vi "Vecto Info JSON.vi"(8 "error in (no error)":errorcluster, 10 "Vecto Info":T1) -> (0 "error out":errorcluster, 2 "JSON string":string)   [LabVIEW 2020, in "Vecto.lvlib" / "InfoController.lvclass"]
uses:
  InfoController.lvclass
  Connection Type.ctl
  Vecto.lvlib
  Connection Info.ctl
  Vecto Info.ctl
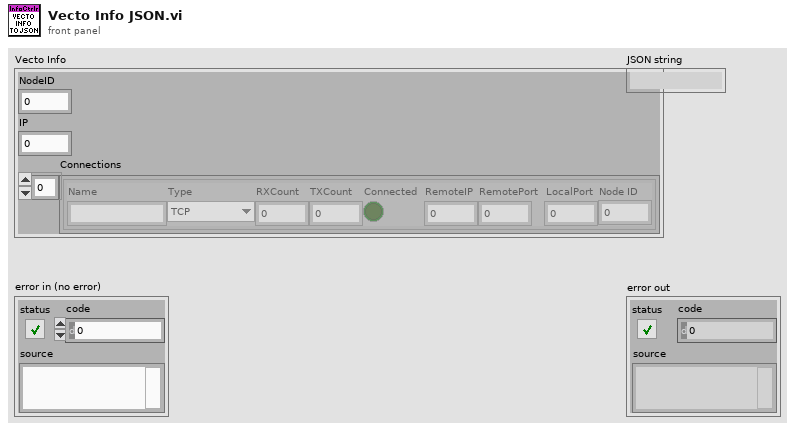
[diagram p1: front panel]
types:
  T1 = typedef "Vecto.lvlib/Vecto Info.ctl" = cluster{"NodeID":i32, "IP":u32, "Connections":T2[]}
  T2 = typedef "Vecto.lvlib/Connection Info.ctl" = cluster{"Name":string, "Type":T3, "RXCount":i32, "TXCount":i32, "Connected":bool, "RemoteIP":u32, "RemotePort":u16, "LocalPort":u16, "Node ID":u32}
  T3 = typedef "Vecto.lvlib/Connection Type.ctl" = enum16{"TCP", "Telemetry", "Discovery", "HTTP"}
  T4 = cluster{"Name":string, "Type":string, "RXCount":i32, "TXCount":i32, "Connected":bool, "RemoteIP":u32, "RemotePort":u16, "LocalPort":u16}[]
  T5 = cluster{"Name":string, "Type":string, "RXCount":i32, "TXCount":i32, "Connected":bool, "RemoteIP":u32, "RemotePort":u16, "LocalPort":u16}
  T6 = cluster{"NodeID":i32, "IP":u32, "Connections":cluster{"Name":string, "Type":string, "RXCount":i32, "TXCount":i32, "Connected":bool, "RemoteIP":u32, "RemotePort":u16, "LocalPort":u16}[]}
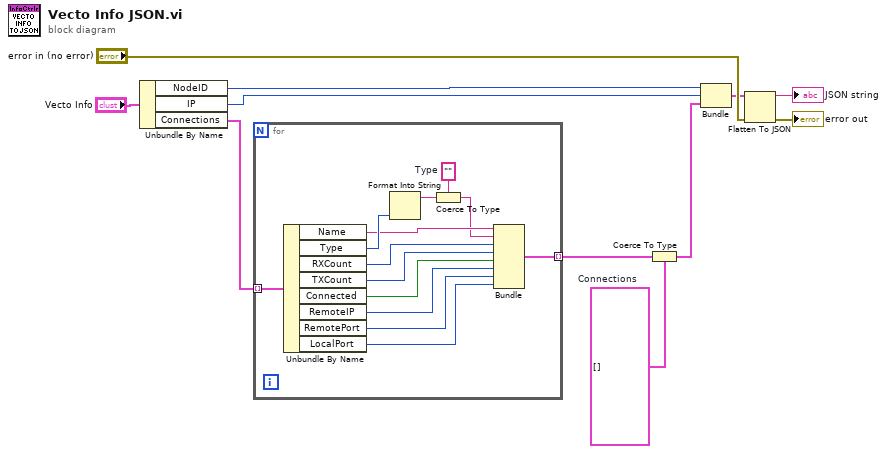
[diagram p0: block diagram]
diagram:
  w1 = T4 []  # Connections
  n1 = Unbundle By Name("Vecto Info") -> ("NodeID"=w10:i32, "IP"=w9:u32, "Connections"=w8:T2[])
  n2 = for {
    tunnel: w8 -> [w24] mode=indexing
    tunnel: [w12] -> w4 mode=indexing
    w21 = ""  # Type
    n3 = Unbundle By Name(w24) -> ("Name"=w20:string, "Type"=w23:T3, "RXCount"=w18:i32, "TXCount"=w17:i32, "Connected"=w16:bool, "RemoteIP"=w15:u32, "RemotePort"=w14:u16, "LocalPort"=w13:u16)
    n4 = Format Into String(w23) -> (resulting string=w22:string)  [unwired: 3 in, 1 out]
    n5 = Coerce To Type(0:w22, 1:w21) -> (2:w19:string)
    n6 = Bundle("Name"=w20, "Type"=w19, "RXCount"=w18, "TXCount"=w17, "Connected"=w16, "RemoteIP"=w15, "RemotePort"=w14, "LocalPort"=w13) -> (w12:T5)  [unwired: 1 in]
  }
  n7 = Coerce To Type(0:w4, 1:w1) -> (2:w3:T4)
  n8 = Bundle("NodeID"=w10, "IP"=w9, "Connections"=w3) -> (w2:T6)  [unwired: 1 in]
  n9 = Flatten To JSON(anything=w2, error in (no error)="error in (no error)") -> (JSON string=→"JSON string":string, 11:→"error out":errorcluster)  [unwired: 1 in]
